vi "_File Manager.vi"(7 "Action":T1, 8 "Error In":errorcluster, 11 "Set Value":variant) -> (0 "Error Out":errorcluster)   [LabVIEW 2014, in "LV-Logger.lvlib"]
uses:
  LV-Logger.lvlib
  _File Manager Action.ctl
  Public/Controls/Message.ctl
  Public/Controls/Tag.ctl
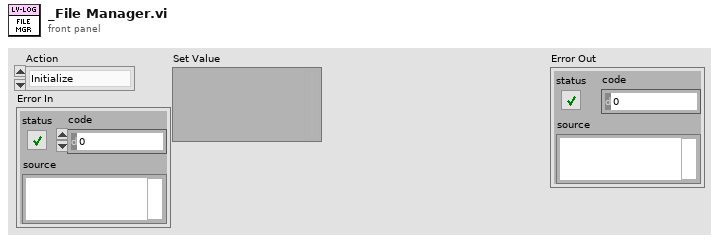
[diagram p1: front panel]
types:
  T1 = typedef "LV-Logger.lvlib/_File Manager Action.ctl" = enum16{"Initialize", "Set File Size Limit", "Set Root Folder", "Set Application Name", "Start", "Write", "Stop", "Shutdown"}
  T2 = typedef "LV-Logger.lvlib/Message.ctl" = cluster{"Time Stamp":timestamp, "Tag":T3, "Source":string, "Text":string}
  T3 = typedef "LV-Logger.lvlib/Tag.ctl" = enum16{"Fatal", "Error", "Warn", "Info", "Debug", "Trace"}
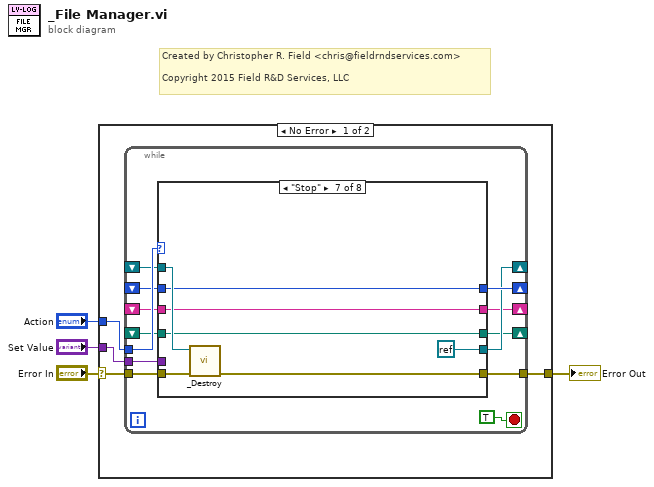
[diagram p0: block diagram]
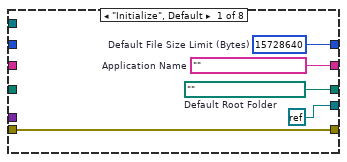
[diagram p2: hidden frame]
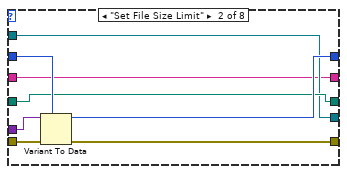
[diagram p3: hidden frame]
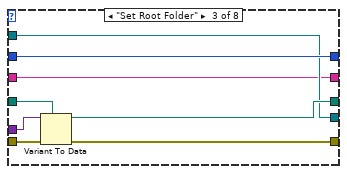
[diagram p4: hidden frame]
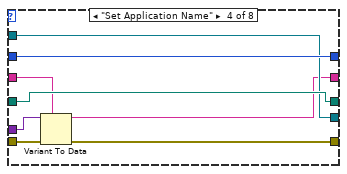
[diagram p5: hidden frame]
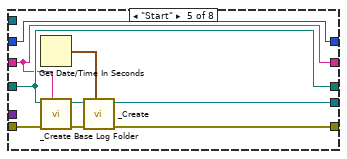
[diagram p6: hidden frame]
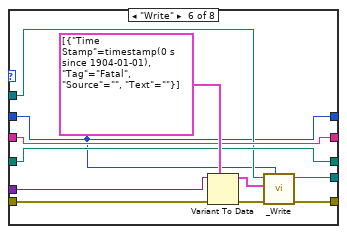
[diagram p7: hidden frame]
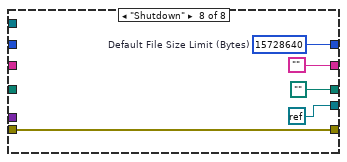
[diagram p8: hidden frame]
diagram:
  # "Created by Christopher R. Field <chris@fieldrndservices.com>\n\nCopyright 2015 Field R&D Services, LLC"
  n1 = case shown="No Error" "Error In" {
    selector: "Error In" -> [w7 w83]
    tunnel: "Action" -> [w8 _]
    tunnel: "Set Value" -> [w6 _]
    tunnel: [w5 w83] -> w1
    frame No Error {
      n2 = while {
        tunnel: w8 -> [w20]
        shift-right: [w19] -> _
        shift-left: _ -> [w14]
        shift-right: [w18] -> _
        shift-left: _ -> [w11]
        shift-right: [w17] -> _
        shift-left: _ -> [w12]
        tunnel: w7 -> [w16]
        tunnel: w6 -> [w15]
        tunnel: [w13] -> w5
        shift-right: [w10] -> _
        shift-left: _ -> [w9]
        stop <- TRUE stop-if-true
        n3 = case shown="\"Stop\"" w20 {
          tunnel: [w26 w31 w42 w50 w59 w62 w72 w78] -> w19
          tunnel: [refnum<k0> refnum w28 w36 w48 w53 w61 refnum<k0> refnum refnum<k0> refnum] -> w18
          tunnel: [w24 w29 w38 w49 w54 w66 w74 path ""] -> w17
          tunnel: w16 -> [w23 w34 w40 w46 w55 w69 w77 w81]
          tunnel: w15 -> [_ w33 w41 w47 _ w70 _ _]
          tunnel: w14 -> [_ w32 w42 w50 w59 w62 w72 _]
          tunnel: [w23 w30 w37 w43 w58 w60 w71 w81] -> w13
          tunnel: w12 -> [_ w29 w39 w49 w54 w66 w74 _]
          tunnel: w11 -> [_ w28 w36 w48 _ w63 w76 _]
          tunnel: [w22 w27 w35 w44 w51 w67 w73 ""] -> w10
          tunnel: w9 -> [_ w27 w35 w45 w51 w67 w73 _]
          frame "Initialize", Default {
            w22 = ""  # Application Name
            w24 = path ""  # Default Root Folder
            w26 = i64 15728640  # Default File Size Limit (Bytes)
          }
          frame "Set File Size Limit" {
            n4 = Variant To Data(error in=w34, type=w32, Variant=w33) -> (data=w31:i64, error out=w30:errorcluster)
          }
          frame "Set Root Folder" {
            n5 = Variant To Data(error in=w40, type=w39, Variant=w41) -> (data=w38:path, error out=w37:errorcluster)
          }
          frame "Set Application Name" {
            n6 = Variant To Data(error in=w46, type=w45, Variant=w47) -> (data=w44:string, error out=w43:errorcluster)
          }
          frame "Start" {
            n7 = Get Date/Time In Seconds() -> (seconds since 1Jan1904=w52:timestamp)
            n8 = call "_Create Base Log Folder.vi"("Application Name"=w51, "Error In"=w55, "Root Folder"=w54) -> ("Error Out"=w56:errorcluster, "Base Log Folder"=w57:path)  [unwired: 7 in]
            n9 = call "_Create.vi"("Start Time Stamp"=w52, "Error In"=w56, "Base Log Folder"=w57) -> ("Error Out"=w58:errorcluster, "Log Out"=w53:refnum<file>)  [unwired: 7 in]
          }
          frame "Write" {
            n10 = Variant To Data(error in=w69, type=T2[] [{"Time Stamp"=timestamp(0 s since 1904-01-01), "Tag"=enum."Fatal", "Source"="", "Text"=""}], Variant=w70) -> (data=w65:T2[], error out=w64:errorcluster)
            n11 = call "_Write.vi"("File Size Limit (Bytes)"=w62, "Error In"=w64, "Messages"=w65, "Log In"=w63) -> ("Error Out"=w60:errorcluster, "Log Out"=w61:refnum<file>)  [unwired: 6 in]
          }
          frame "Stop" {
            n12 = call "_Destroy.vi"("Error In"=w77, "Log In"=w76) -> ("Error Out"=w71:errorcluster)  [unwired: 8 in, 1 out]
          }
          frame "Shutdown" {
            w78 = i64 15728640  # Default File Size Limit (Bytes)
          }
        }
      }
    }
    frame Error {
    }
  }
  "Error Out" <- w1
